vi "GetType.vi"(8 "error in (no error)":errorcluster, 11 "Configure Meas Complete Dest [MP] Msg":refnum<class "Configure Meas Complete Dest [MP] Msg.lvclass">) -> (0 "error out":errorcluster, 2 "Data Sample":variant, 3 "Configure Meas Complete Dest [MP] Msg":refnum<class "Configure Meas Complete Dest [MP] Msg.lvclass">)   [LabVIEW 2016, in "CS++DMM.lvlib" / "Configure Meas Complete Dest [MP] Msg.lvclass"]
uses:
  Configure Meas Complete Dest [MP] Msg.lvclass
  Configure Meas Complete Dest [MP] Msg.lvclass/Configure Meas Complete Dest [MP] Msg.ctl
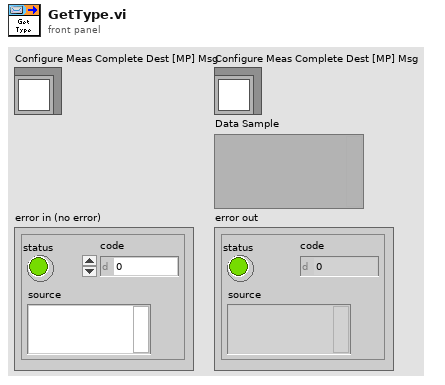
[diagram p1: front panel]
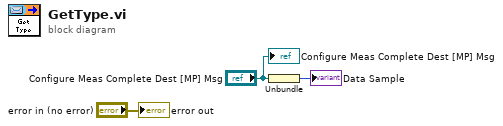
[diagram p0: block diagram]
diagram:
  n1 = Unbundle("Configure Meas Complete Dest [MP] Msg") -> (→"Data Sample":i32)
  "error out" <- "error in (no error)"
  "Configure Meas Complete Dest [MP] Msg" <- "Configure Meas Complete Dest [MP] Msg"
